vi "DrawCircle2.vi"(1 "Color":u32(colorbox)=6618880, 3 "Fitted Circle (左圆)":T1 {"Average SNR (dB)" format="%.2f"; "Average Strength" format="%.2f"; "Roundness (Real-World)" format="%.2f"; "Radius (Real-World)" format="%.2f"; "Center (Real-World)"."Y" format="%.2f"; "Center (Real-World)"."X" format="%.2f"; "Radius (Pixels)" format="%.2f"; "Center (Pixels)"."Y" format="%.2f"; "Center (Pixels)"."X" format="%.2f"}, 4 "Img in":T2) -> (0 "Img out":T2)   [LabVIEW 2014]
uses:
  <vilib>/vision/Image Controls.llb/IMAQ Image.ctl
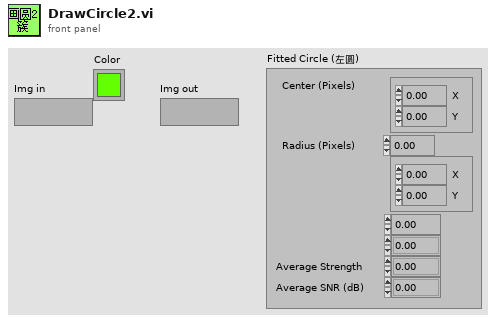
[diagram p1: front panel]
types:
  T1 = cluster{"Center (Pixels)":cluster{"X":sgl, "Y":sgl}, "Radius (Pixels)":dbl, "Center (Real-World)":cluster{"X":sgl, "Y":sgl}, "Radius (Real-World)":dbl, "Roundness (Real-World)":dbl, "Average Strength":dbl, "Average SNR (dB)":dbl}
  T2 = typedef "IMAQ Image.ctl" = refnum<image>
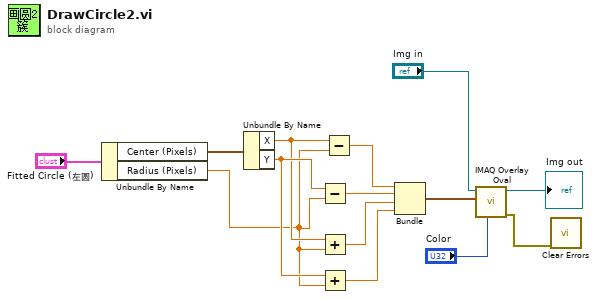
[diagram p0: block diagram]
diagram:
  n1 = Unbundle By Name("Fitted Circle (左圆)") -> ("Center (Pixels)"=w3:cluster{"X":sgl, "Y":sgl}, "Radius (Pixels)"=w2:dbl)
  n2 = Unbundle By Name(w3) -> ("X"=w6:sgl, "Y"=w7:sgl)
  n3 = Subtract(x=w7, y=w2) -> (x-y=w9:dbl)
  n4 = Add(x=w6, y=w2) -> (x+y=w10:dbl)
  n5 = Add(x=w7, y=w2) -> (x+y=w11:dbl)
  n6 = Subtract(x=w6, y=w2) -> (x-y=w8:dbl)
  n7 = Bundle(w8, w9, w10, w11) -> (w12:cluster{dbl, dbl, dbl, dbl})  [unwired: 1 in]
  n8 = call "IMAQ Overlay Oval"("Color"="Color", "Bounding Rectangle"=w12, "Image"="Img in") -> ("error out"=w1:errorcluster, "Image Out"=→"Img out":T2)  [unwired: 7 in]
  n9 = call <vilib>:"Clear Errors.vi"("error in (no error)"=w1) -> ()  [unwired: 5 in, 2 out]
